vi "900x 9870 DMA Read (Sub).vi"(8 "error in":errorcluster, 9 "Number of Bytes":i32, 11 "FPGA In":T1) -> (0 "error out":errorcluster, 1 "Byte Count":u32, 2 "Read Bytes":string, 3 "FPGA Out":T1, 4 "Timed Out":bool, 6 "FPGA Error":errorcluster)   [LabVIEW 2012]
uses:
  900x DMA FPGA Reference.ctl
  FPGA Function.ctl
  <vilib>/Utility/error.llb/Error Cluster From Error Code.vi
  <vilib>/rvi/errors/niLvFpgaAdjustHostInterfaceError.vi
  <vilib>/rvi/interface/nirviReadWriteControl/nirviReadWriteControl.xnode
  FPGA Bitfiles/NI-987xSerialLoo_FPGATarget2_9870InterfaceDMA_83BB861F.lvbitx
  Program Files (x86)/National Instruments/LabVIEW 2012/examples/CompactRIO/Module Specific/NI 987x/Serial Loopback/VIs/9870 Interface DMA Rd (FPGA).vi
  <vilib>/rvi/interface/nirviMethod/nirviMethod.xnode
  NiFpgaLv.dll
  <vilib>/FPGAPlugInAG/cRIO-9101/niLvFpga_AcknowledgeIrq_cRIO-9101.vi
  <vilib>/rvi/interface/nirviMethod/StockFPGA_InlinedMethodWaitForSingleIRQ.vi
  <vilib>/FPGAPlugInAG/cRIO-9101/niLvFpga_WaitOnIrq_cRIO-9101.vi
  <vilib>/FPGAPlugInAG/cRIO-9101/niLvFpga_ReadFifo_cRIO-9101.vi
  <vilib>/rvi/errors/niLvFpgaMergeErrorWithErrorCode.vi
panel:
  # "Input"
  # "Output"
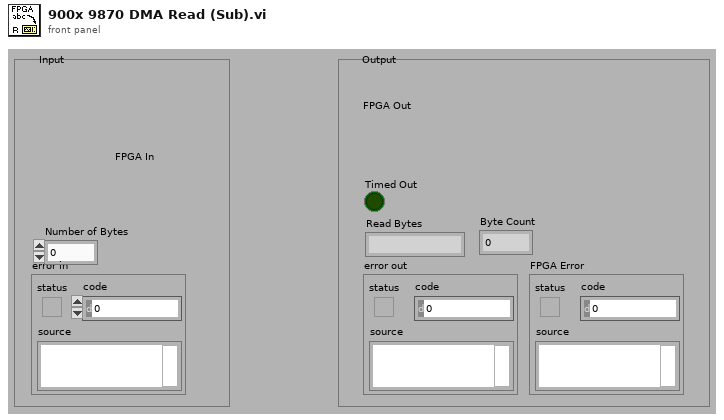
[diagram p1: front panel]
types:
  T1 = typedef "900x DMA FPGA Reference.ctl" = refnum<k20>
  T2 = typedef "FPGA Function.ctl" = enum16{"Do Nothing", "Write", "Read"}
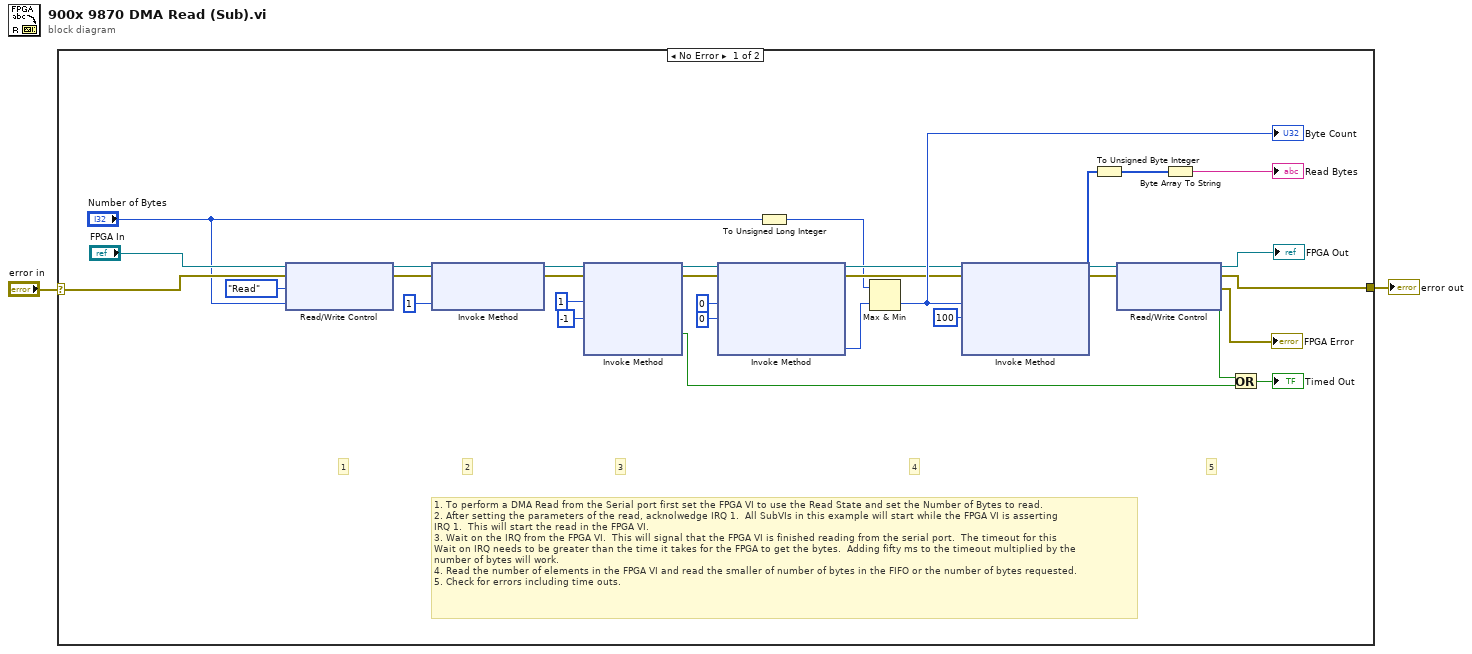
[diagram p0: block diagram]
diagram:
  n1 = case shown="No Error" "error in" {
    selector: "error in" -> [w5 w35]
    tunnel: [w34 w35] -> w2
    frame No Error {
      # "1. To perform a DMA Read from the Serial port first set the FPGA VI to use the Read State and set the Number of Bytes to read.\n2. After setting the parameters of the read, acknolwedge IRQ 1.  All SubVIs in this example will start while the FPGA VI is asserting \nIRQ 1.  This will start the read in the FPGA VI.\n3. Wait on the IRQ from the FPGA VI.  This will signal that the FPGA VI is finished reading from the serial port.  The timeout for this \nWait on IRQ needs to be greater than the time it takes for the FPGA to get the bytes.  Adding fifty ms to the timeout multiplied by the \nnumber of bytes will work.\n4. Read the number of elements in the FPGA VI and read the smaller of number of bytes in the FIFO or the number of bytes requested.\n5. Check for errors including time outs."
      # "5"
      # "4"
      # "3"
      # "2"
      # "1"
      n2 = xnode "Read/Write Control"("FPGA VI Reference In"="FPGA In", "error in"=w5, "Op Control"=FPGA_Function."Read", "Number of Bytes"="Number of Bytes") -> ("FPGA VI Reference Out"=w30:T1, "error out"=w29:errorcluster)
      n3 = xnode "Invoke Method"("FPGA VI Reference In"=w30, "error in"=w29, "IRQ Number(s)"=1) -> ("FPGA VI Reference Out"=w22:T1, "error out"=w21:errorcluster)
      n4 = xnode "Invoke Method"("FPGA VI Reference In"=w22, "error in"=w21, "IRQ Number(s)"=1, "Timeout (ms)"=-1) -> ("FPGA VI Reference Out"=w9:T1, "error out"=w8:errorcluster, "Timed Out"=w17:bool)  [unwired: 1 out]
      n5 = xnode "Invoke Method"("FPGA VI Reference In"=w9, "error in"=w8, "Number of Elements"=u32 0, "Timeout (ms)"=0) -> ("FPGA VI Reference Out"=w26:T1, "error out"=w25:errorcluster, "Elements Remaining"=w24:u32)  [unwired: 1 out]
      n6 = To Unsigned Long Integer(number="Number of Bytes") -> (unsigned 32bit integer=w10:u32)
      n7 = Max & Min(x=w10, y=w24) -> (min(x,y)=w32:u32)  [unwired: 1 out]
      "Byte Count" <- w32
      n8 = xnode "Invoke Method"("FPGA VI Reference In"=w26, "error in"=w25, "Number of Elements"=w32, "Timeout (ms)"=100) -> ("FPGA VI Reference Out"=w28:T1, "error out"=w27:errorcluster, "Data"=w18:u32[])  [unwired: 1 out]
      n9 = To Unsigned Byte Integer(number=w18) -> (unsigned 8bit integer=w14:u8[])
      n10 = xnode "Read/Write Control"("FPGA VI Reference In"=w28, "error in"=w27) -> ("FPGA VI Reference Out"=→"FPGA Out":T1, "error out"=w34:errorcluster, "error out"=→"FPGA Error":errorcluster, "Timed Out Read"=w7:bool)
      n11 = Byte Array To String(unsigned byte array=w14) -> (string=→"Read Bytes":string)
      n12 = Or(x=w7, y=w17) -> (x .or. y?=→"Timed Out":bool)
    }
    frame Error {
    }
  }
  "error out" <- w2
